vi "Add Connection.vi"(8 "error in (no error)":errorcluster, 9 "channel 2":string, 10 "channel 1":string, 11 "SLSC Switch in":refnum<class "SLSC Switch.lvclass">) -> (0 "error out":errorcluster, 3 "SLSC Switch out":refnum<class "SLSC Switch.lvclass">)   [LabVIEW 2017, in "SLSC Switch.lvlib" / "SLSC Switch.lvclass"]
uses:
  SLSC Switch.lvclass
  Controls/Connection.ctl
  SLSC Switch.lvclass/SLSC Switch.ctl
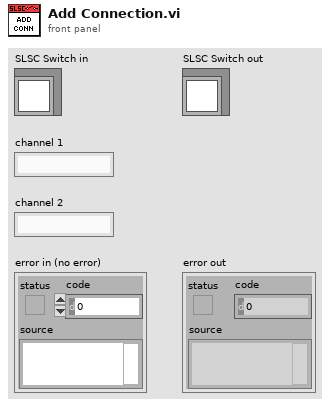
[diagram p1: front panel]
types:
  T1 = typedef "SLSC Switch.lvlib/SLSC Switch.lvclass/Connection.ctl" = cluster{"channel 1":string, "channel 2":string}
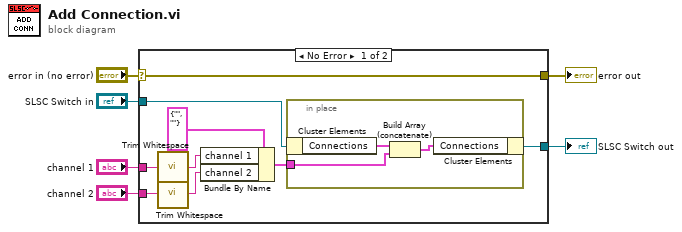
[diagram p0: block diagram]
diagram:
  n1 = case shown="No Error" "error in (no error)" {
    selector: "error in (no error)" -> [w15 w20]
    tunnel: [w15 w20] -> w5
    tunnel: [w13 w19] -> w3
    tunnel: "SLSC Switch in" -> [w14 w19]
    tunnel: "channel 1" -> [w10 _]
    tunnel: "channel 2" -> [w8 _]
    frame No Error {
      n2 = call <vilib>:"Trim Whitespace.vi"("string"=w10) -> ("trimmed string"=w9:string)  [unwired: 1 in]
      n3 = call <vilib>:"Trim Whitespace.vi"("string"=w8) -> ("trimmed string"=w7:string)  [unwired: 1 in]
      n4 = Bundle By Name(cluster=T1 {"channel 1"="", "channel 2"=""} ("connections"), "channel 1"=w9, "channel 2"=w7) -> (w11:T1)
      n5 = in-place {
        in-place-border: w11 -> [w17]
        n6 = in-place-cluster #1(w14) -> ("Connections"=w18:T1[])
        n7 = Build Array (concatenate)(w18, w17) -> (w16:T1[])
        n8 = in-place-cluster #1("Connections"=w16) -> (w13:refnum<class "SLSC Switch.lvclass">)
      }
    }
    frame Error {
    }
  }
  "error out" <- w5
  "SLSC Switch out" <- w3
